vi "photosensor.vi"() -> ()   [LabVIEW 2018]
panel:
  out "Avg Voltage":dbl=1000.0 format="%0.2f"
  in  "stop":bool
  out "error out":errorcluster
  in  "error in":errorcluster
  in  "Number of Samples":i32=100
  in  "Sample Rate":dbl=1000.0
  in  "Min Voltage":dbl=-5.0
  in  "Max Voltage":dbl=5.0
  in  "Physical Channel":tag="Dev1/ai0"
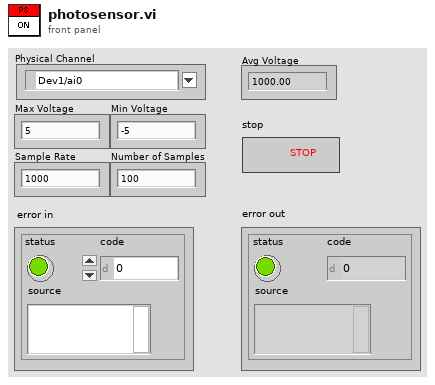
[diagram p1: front panel]
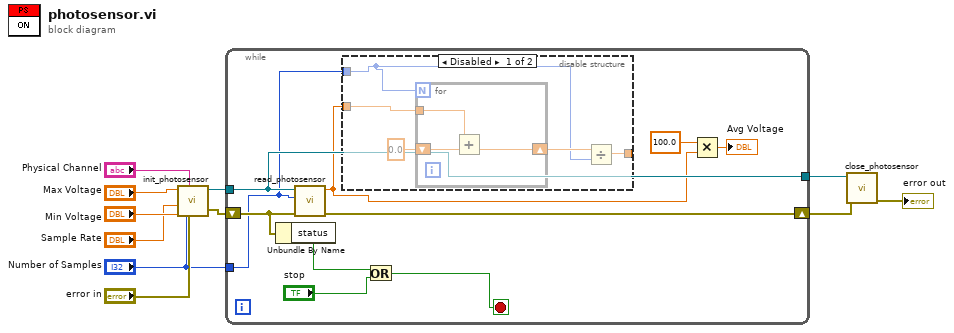
[diagram p0: block diagram]
diagram:
  n1 = call "init_photosensor.vi"("error in"="error in", "Physical Channel"="Physical Channel", "Number of Samples"="Number of Samples", "Sample Rate"="Sample Rate", "Min Voltage"="Min Voltage", "Max Voltage"="Max Voltage") -> ("task out"=w3:refnum<k21>, "error out"=w5:errorcluster)  [unwired: 4 in]
  n2 = while {
    tunnel: w3 -> [w16]
    shift-right: [w21] -> w4
    shift-left: w5 -> [w20]
    tunnel: [w16] -> w2
    tunnel: "Number of Samples" -> [w15]
    stop <- w19 stop-if-true
    n3 = Unbundle By Name(w20) -> ("status"=w17:bool)
    n4 = call "read_photosensor.vi"("error in"=w20, "number of samples"=w15, "task/channels in"=w16) -> ("error out"=w21:errorcluster, "Avg Voltage"=w14:dbl)  [unwired: 6 in]
    n5 = disable-structure shown="Disabled" {
      disable-tunnel: [w24 _] -> _
      disable-tunnel: w14 -> [w23 _]
      disable-tunnel: w15 -> [w22 _]
      frame Disabled {
        n6 = for {
          N: w22 -> [_]
          tunnel: w23 -> [w29]
          shift-right: [w28] -> w25
          shift-left: 0.0 -> [w27]
          n7 = Add(x=w29, y=w27) -> (x+y=w28:dbl)
        }
        n8 = Divide(x=w25, y=w22) -> (x/y=w24:dbl)
      }
      frame Enabled {
      }
    }
    n9 = Or(x=w17, y="stop") -> (x .or. y?=w19:bool)
    n10 = Multiply(x=100.0, y=w14) -> (x*y=→"Avg Voltage":dbl)
  }
  n11 = call "close_photosensor.vi"("error in"=w4, "task/channels in"=w2) -> ("error out"=→"error out":errorcluster)  [unwired: 9 in]
